vi "LEDCheck.vi"(8 "error in (no error)":errorcluster, 10 "Cluster in":T2, 11 "Enum in":T1=enum."Idle") -> (0 "error out":errorcluster, 2 "Cluster":T2, 3 "Enum out":T1=enum."Idle")   [LabVIEW 2018]
uses:
  Type_Def/Type_Def Actuator Controls.ctl
  Type_Def/Type_Def ControlState.ctl
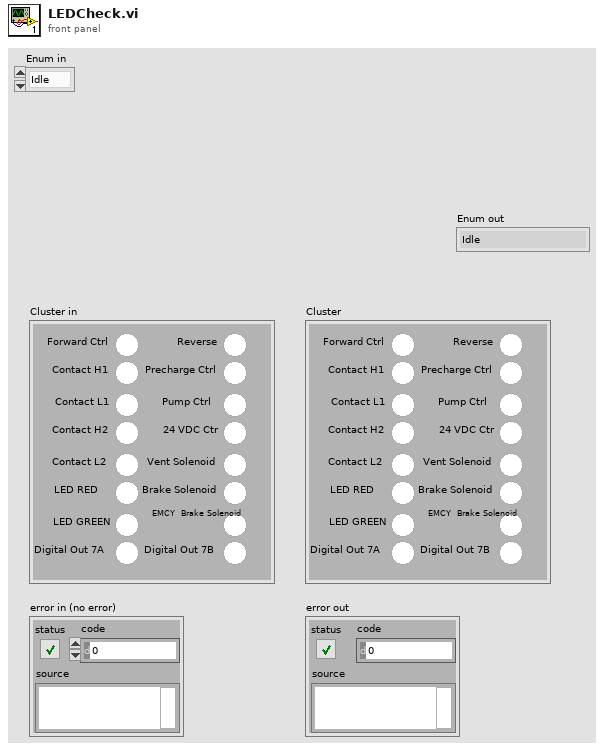
[diagram p1: front panel]
types:
  T1 = typedef "Type_Def ControlState.ctl" = enum16{"Blank", "Systems Check", "Idle", "Ready", "Pushing", "CrawlingPrecharge", "Braking", "Fault", "Boot Up", "Unpowered", "Crawling", "Shutdown", "Service Push", "Service Wait", "Vent", "Precharge"}
  T2 = typedef "Type_Def Actuator Controls.ctl" = cluster{"Reverse ":bool, "Precharge Ctrl":bool, "Pump Ctrl":bool, "24 VDC Ctr":bool, "Vent Solenoid":bool, "Brake Solenoid":bool, "EMCY  Brake Solenoid":bool, "Digital Out 7B ":bool, "Forward Ctrl":bool, "Contact H1":bool, "Contact L1":bool, "Contact H2":bool, "Contact L2 ":bool, "LED RED":bool, "LED GREEN":bool, " Digital Out 7A":bool}
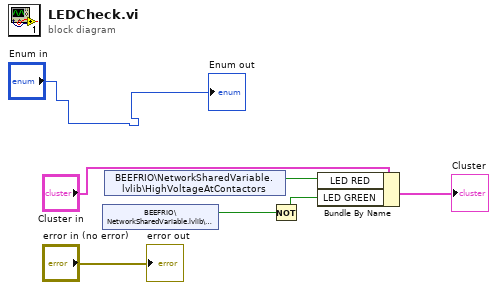
[diagram p0: block diagram]
diagram:
  n1 = shared-variable "BEEFRIO\\NetworkSharedVariable.lvlib\\IsolationFault"() -> (w3:bool)  [unwired: 1 in, 1 out]
  n2 = shared-variable "BEEFRIO\\NetworkSharedVariable.lvlib\\HighVoltageAtContactors"() -> (w4:bool)  [unwired: 1 in, 1 out]
  n3 = Not(x=w3) -> (.not. x?=w2:bool)
  n4 = Bundle By Name(cluster="Cluster in", "LED RED"=w4, "LED GREEN"=w2) -> (→"Cluster":T2)
  "error out" <- "error in (no error)"
  "Enum out" <- "Enum in"
